vi "Read Calibrations + Settings 2016.vi"   [LabVIEW 2015]
uses:
  Global Variables/Calibrations.vi
  Global Variables/Settings.vi
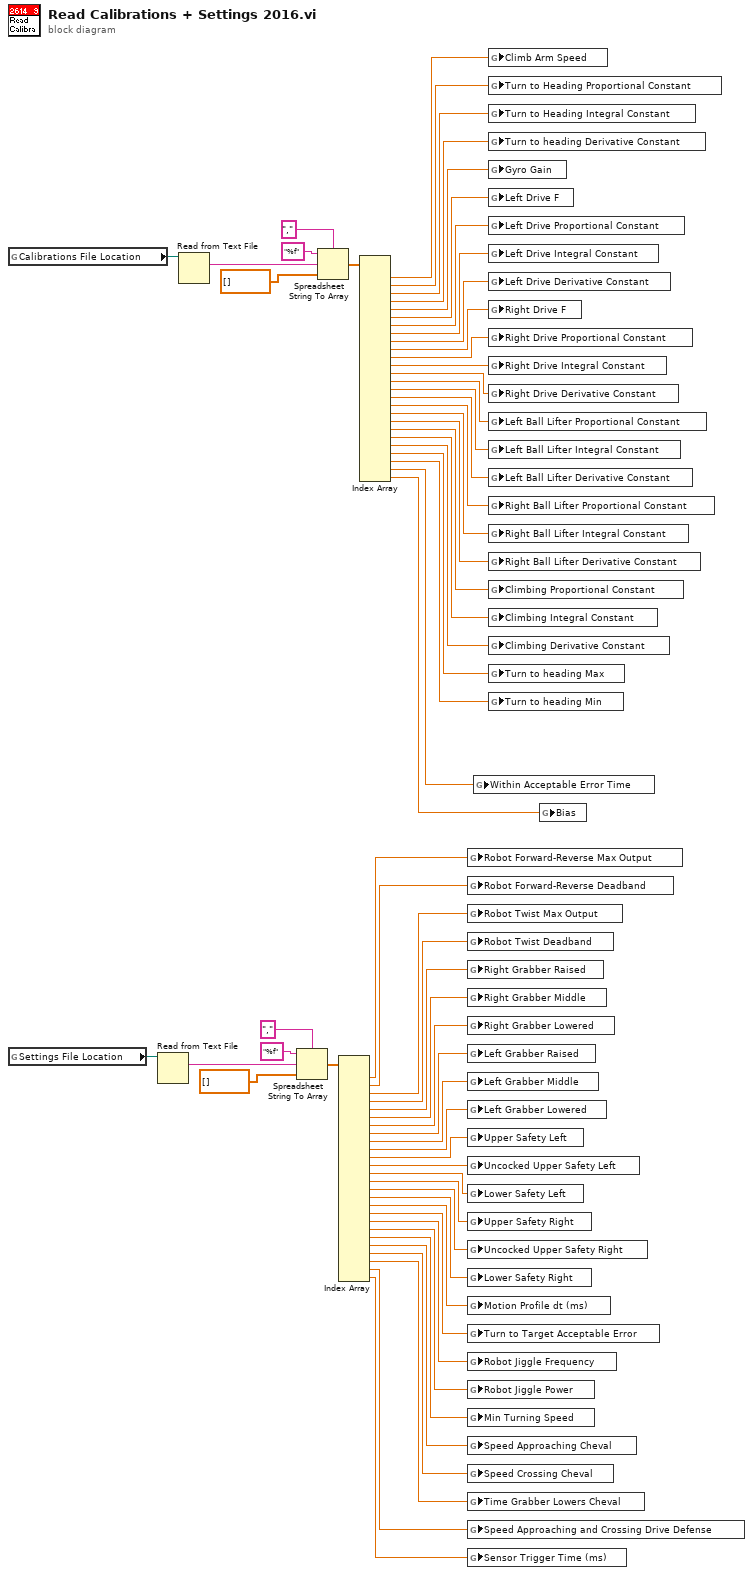
[diagram p0: block diagram]
diagram:
  n1 = global read "Calibrations.vi" "Calibrations File Location"() -> (w60:path)
  n2 = global read "Settings.vi" "Settings File Location"() -> (w55:path)
  n3 = Read from Text File(file (use dialog)=w55) -> (text=w59:string)  [unwired: 3 in, 3 out]
  n4 = Read from Text File(file (use dialog)=w60) -> (text=w64:string)  [unwired: 3 in, 3 out]
  n5 = Spreadsheet String To Array(delimiter (Tab)=",", format string="%f", spreadsheet string=w59, array type (2D Dbl)=dbl[] []) -> (array=w18:dbl[])
  n6 = Spreadsheet String To Array(delimiter (Tab)=",", format string="%f", spreadsheet string=w64, array type (2D Dbl)=dbl[] []) -> (array=w54:dbl[])
  n7 = Index Array(array=w18) -> (element #1=w35:dbl, element #2=w34:dbl, element #3=w27:dbl, element #4=w33:dbl, element #5=w32:dbl, element #6=w31:dbl, element #7=w30:dbl, element #8=w29:dbl, element #9=w28:dbl, element #10=w26:dbl, element #11=w25:dbl, element #12=w24:dbl, element #13=w23:dbl, element #14=w22:dbl, element #15=w21:dbl, element #16=w20:dbl, element #17=w19:dbl, element #18=w12:dbl, element #19=w11:dbl, element #20=w10:dbl, element #21=w9:dbl, element #22=w7:dbl, element #23=w6:dbl, element #24=w5:dbl, element #25=w4:dbl, element #26=w3:dbl)  [unwired: 26 in]
  n8 = Index Array(array=w54) -> (element #1=w14:dbl, element #2=w53:dbl, element #3=w52:dbl, element #4=w36:dbl, element #5=w51:dbl, element #6=w50:dbl, element #7=w48:dbl, element #8=w49:dbl, element #9=w47:dbl, element #10=w46:dbl, element #11=w43:dbl, element #12=w45:dbl, element #13=w44:dbl, element #14=w42:dbl, element #15=w41:dbl, element #16=w40:dbl, element #17=w39:dbl, element #18=w38:dbl, element #19=w37:dbl, element #20=w15:dbl, element #21=w16:dbl, element #22=w17:dbl, element #23=w13:dbl, element #24=w8:dbl, element #25=w2:dbl, element #26=w1:dbl)  [unwired: 26 in]
  n9 = global write "Settings.vi" "Robot Forward-Reverse Max Output"(w35) -> ()
  n10 = global write "Settings.vi" "Robot Forward-Reverse Deadband"(w34) -> ()
  n11 = global write "Settings.vi" "Robot Twist Max Output"(w27) -> ()
  n12 = global write "Settings.vi" "Robot Twist Deadband"(w33) -> ()
  n13 = global write "Settings.vi" "Right Grabber Raised"(w32) -> ()
  n14 = global write "Settings.vi" "Right Grabber Middle"(w31) -> ()
  n15 = global write "Settings.vi" "Right Grabber Lowered"(w30) -> ()
  n16 = global write "Settings.vi" "Left Grabber Raised"(w29) -> ()
  n17 = global write "Settings.vi" "Left Grabber Middle"(w28) -> ()
  n18 = global write "Settings.vi" "Left Grabber Lowered"(w26) -> ()
  n19 = global write "Settings.vi" "Upper Safety Left"(w25) -> ()
  n20 = global write "Settings.vi" "Uncocked Upper Safety Left"(w24) -> ()
  n21 = global write "Settings.vi" "Lower Safety Left"(w23) -> ()
  n22 = global write "Settings.vi" "Upper Safety Right"(w22) -> ()
  n23 = global write "Settings.vi" "Uncocked Upper Safety Right"(w21) -> ()
  n24 = global write "Settings.vi" "Lower Safety Right"(w20) -> ()
  n25 = global write "Settings.vi" "Motion Profile dt (ms)"(w19) -> ()
  n26 = global write "Settings.vi" "Turn to Target Acceptable Error"(w12) -> ()
  n27 = global write "Settings.vi" "Robot Jiggle Frequency"(w11) -> ()
  n28 = global write "Settings.vi" "Robot Jiggle Power"(w10) -> ()
  n29 = global write "Settings.vi" "Min Turning Speed"(w9) -> ()
  n30 = global write "Settings.vi" "Speed Approaching Cheval"(w7) -> ()
  n31 = global write "Settings.vi" "Speed Crossing Cheval"(w6) -> ()
  n32 = global write "Settings.vi" "Time Grabber Lowers Cheval"(w5) -> ()
  n33 = global write "Settings.vi" "Speed Approaching and Crossing Drive Defense"(w4) -> ()
  n34 = global write "Settings.vi" "Sensor Trigger Time (ms)"(w3) -> ()
  n35 = global write "Calibrations.vi" "Within Acceptable Error Time"(w2) -> ()
  n36 = global write "Calibrations.vi" "Climb Arm Speed"(w14) -> ()
  n37 = global write "Calibrations.vi" "Turn to Heading Proportional Constant"(w53) -> ()
  n38 = global write "Calibrations.vi" "Turn to Heading Integral Constant"(w52) -> ()
  n39 = global write "Calibrations.vi" "Turn to heading Derivative Constant"(w36) -> ()
  n40 = global write "Calibrations.vi" "Gyro Gain"(w51) -> ()
  n41 = global write "Calibrations.vi" "Left Drive F"(w50) -> ()
  n42 = global write "Calibrations.vi" "Left Drive Proportional Constant"(w48) -> ()
  n43 = global write "Calibrations.vi" "Left Drive Integral Constant"(w49) -> ()
  n44 = global write "Calibrations.vi" "Left Drive Derivative Constant"(w47) -> ()
  n45 = global write "Calibrations.vi" "Right Drive F"(w46) -> ()
  n46 = global write "Calibrations.vi" "Right Drive Proportional Constant"(w43) -> ()
  n47 = global write "Calibrations.vi" "Right Drive Integral Constant"(w45) -> ()
  n48 = global write "Calibrations.vi" "Right Drive Derivative Constant"(w44) -> ()
  n49 = global write "Calibrations.vi" "Left Ball Lifter Proportional Constant"(w42) -> ()
  n50 = global write "Calibrations.vi" "Left Ball Lifter Integral Constant"(w41) -> ()
  n51 = global write "Calibrations.vi" "Left Ball Lifter Derivative Constant"(w40) -> ()
  n52 = global write "Calibrations.vi" "Right Ball Lifter Proportional Constant"(w39) -> ()
  n53 = global write "Calibrations.vi" "Right Ball Lifter Integral Constant"(w38) -> ()
  n54 = global write "Calibrations.vi" "Right Ball Lifter Derivative Constant"(w37) -> ()
  n55 = global write "Calibrations.vi" "Climbing Proportional Constant"(w15) -> ()
  n56 = global write "Calibrations.vi" "Climbing Integral Constant"(w16) -> ()
  n57 = global write "Calibrations.vi" "Climbing Derivative Constant"(w17) -> ()
  n58 = global write "Calibrations.vi" "Turn to heading Max"(w13) -> ()
  n59 = global write "Calibrations.vi" "Turn to heading Min"(w8) -> ()
  n60 = global write "Calibrations.vi" "Bias"(w1) -> ()
